vi "drotg - Givens Rotation Parameters (DBL).vi"(10 "y":dbl, 11 "x":dbl) -> (0 "error":i32, 2 "s":dbl, 3 "c":dbl, 4 "z":dbl, 5 "r":dbl)   [LabVIEW 2017, in "NI_AALBLAS.lvlib"]
doc: "Creates the parameters used in the rot - Givens Rotation VI."
uses:
  NI_AALBLAS.lvlib
  lvblas.dll
panel:
  # "{"
  # "-s*x+c*y=0"
  # "c*x+s*y=r"
  # "c +s =1"
  # "2"
  # "2"
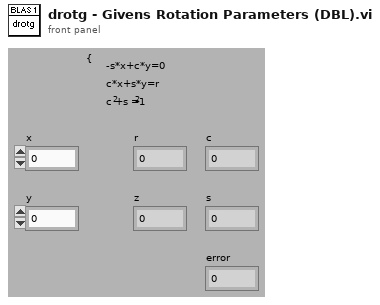
[diagram p1: front panel]
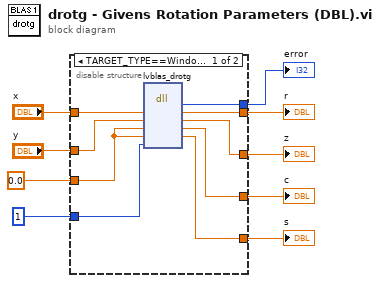
[diagram p0: block diagram]
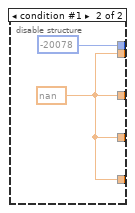
[diagram p2: hidden frame]
diagram:
  n1 = disable-structure shown="TARGET_TYPE==Windows||TARGET_TYPE==Unix||TARGET_TYPE==RT||TARGET_TYPE==Mac" {
    disable-tunnel: [w18 -20078] -> w9
    disable-tunnel: [w17 w19] -> w6
    disable-tunnel: [w16 w19] -> w5
    disable-tunnel: "x" -> [w15 _]
    disable-tunnel: "y" -> [w14 _]
    disable-tunnel: [w13 w19] -> w4
    disable-tunnel: [w12 w19] -> w3
    disable-tunnel: 1 -> [w11 _]
    disable-tunnel: 0.0 -> [w10 _]
    frame condition #0 (active) {
      n2 = dll-call lib="C:/Program Files/National Instruments/LabVIEW 2017/resource/lvblas.*" fn="lvblas_drotg" ("CBLAS.dll:DotProdH")("x"=w15, "y"=w14, "c"=w10, "s"=w10, "check"=w11) -> ("error"=w18:i32, "x"=w17:dbl, "y"=w16:dbl, "c"=w13:dbl, "s"=w12:dbl)  [unwired: 4 in, 2 out]
    }
    frame condition #1 {
      w19 = nan
    }
  }
  "error" <- w9
  "c" <- w4
  "s" <- w3
  "r" <- w6
  "z" <- w5
